vi "Save_current_setup.vi"(3 "Save New File?":bool, 5 "Folder":path) -> (0 "Cancelled?":bool, 1 "Saved filepath":path, 2 "Current Setup":path)   [LabVIEW 2010]
panel:
  in  "Cancel Button":bool
  in  "OK":bool
  out "Existing file names":string[](array[string])
  in  "New setup filename":string
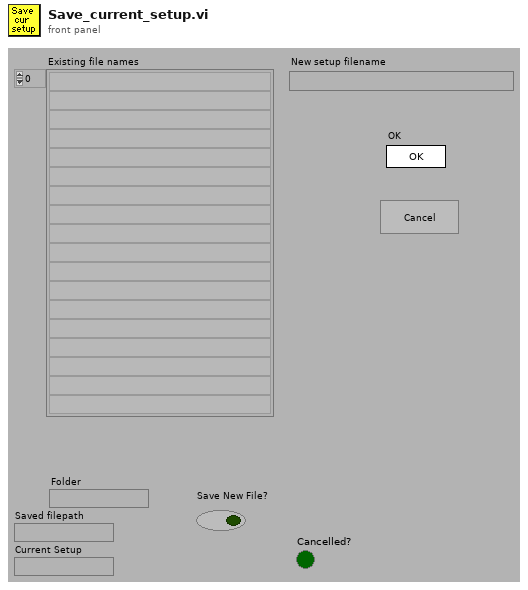
[diagram p1: front panel]
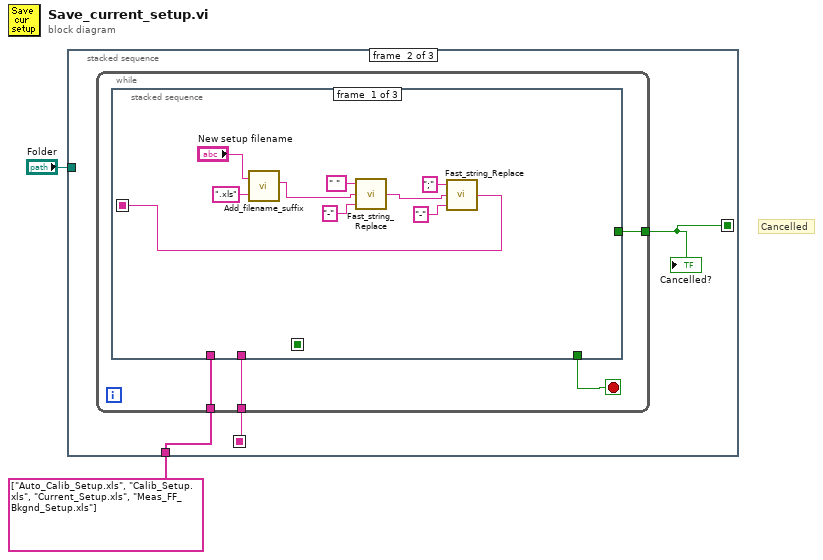
[diagram p0: block diagram]
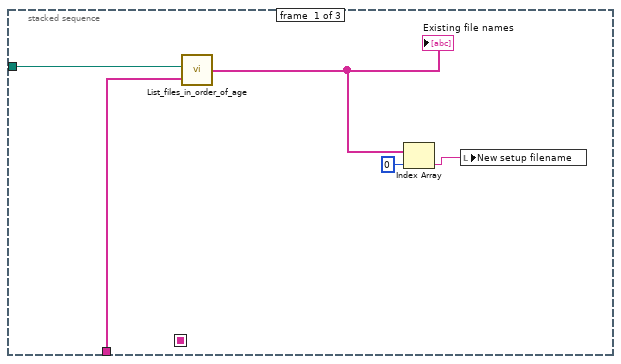
[diagram p2: hidden frame]
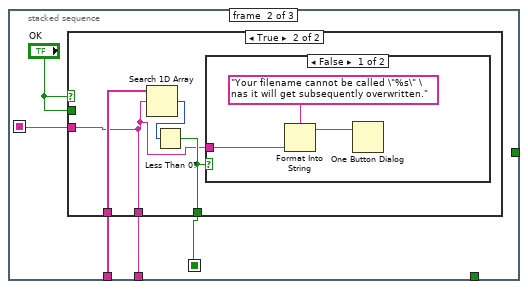
[diagram p3: hidden frame]
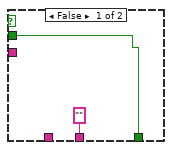
[diagram p4: hidden frame]
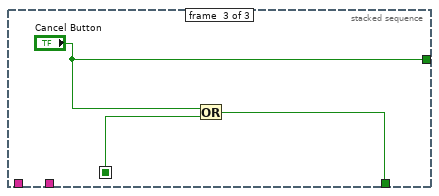
[diagram p6: hidden frame]
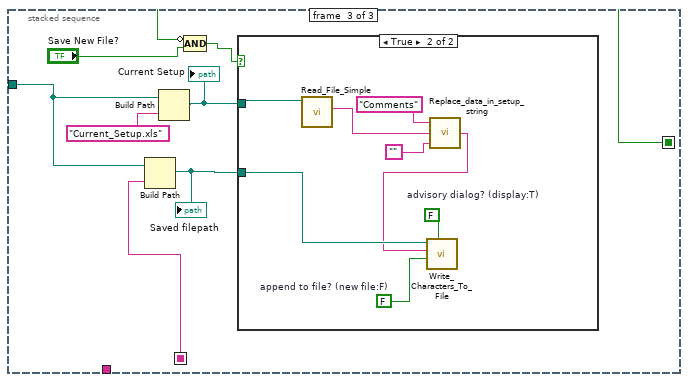
[diagram p7: hidden frame]
diagram:
  # "Cancelled"
  n1 = stacked-sequence {
    seq-local: [_ w10 _] -> [_ _ w47]
    seq-local: [_ w9 _] -> [_ _ w43]
    tunnel: "Folder" -> [w7 _ w46]
    tunnel: string[] ["Auto_Calib_Setup.xls", "Calib_Setup.xls", "Current_Setup.xls", "Meas_FF_Bkgnd_Setup.xls"] ("file names") -> [w6 w8 _]
    frame #0 {
      n2 = call "List_files_in_order_of_age.vi"("Files to Hide"=w6, "Folder"=w7) -> ("file names"=w5:string[])
      "Existing file names" <- w5
      n3 = Index Array(array=w5, index=0) -> (element=w3:string)
      n4 = local write "New setup filename"(w3) -> ()
    }
    frame #1 {
      n5 = while {
        tunnel: [w14] -> w10
        tunnel: [w12] -> w9
        tunnel: w8 -> [w11]
        stop <- w13 stop-if-true
        n6 = stacked-sequence {
          seq-local: [w15 _ _] -> [_ w28 _]
          seq-local: [_ w26 _] -> [_ _ w40]
          tunnel: [_ w27 _] -> w14
          tunnel: [_ _ w39] -> w13
          tunnel: [_ _ "Cancel Button"] -> w12
          tunnel: w11 -> [_ w24 _]
          frame #0 {
            n7 = call "Add_filename_suffix.vi"("Filename"="New setup filename", "Suffix to add"=".xls") -> ("Filename out"=w20:string)  [unwired: 3 out]
            n8 = call "Fast_string_Replace.vi"("Replace match with:"="-", "Input String"=w20, "regular expression"=" ") -> ("Output String"=w16:string)  [unwired: 2 out]
            n9 = call "Fast_string_Replace.vi"("Replace match with:"="-", "Input String"=w16, "regular expression"=";") -> ("Output String"=w15:string)  [unwired: 2 out]
          }
          frame #1 {
            n10 = case shown="True" "OK" {
              tunnel: w28 -> [_ w31]
              tunnel: [w29 w32] -> w26
              tunnel: ["" ("File name only") w31] -> w27
              tunnel: "OK" -> [w29 _]
              tunnel: w24 -> [_ w34]
              frame False {
              }
              frame True {
                n11 = Search 1D Array(1D array=w34, element=w31) -> (index of element=w33:i32)  [unwired: 1 out]
                n12 = Less Than 0?(x=w33) -> (x < 0?=w32:bool)
                n13 = case shown="False" w32 {
                  tunnel: w31 -> [w36 _]
                  frame False {
                    n14 = Format Into String(format string="Your filename cannot be called \"%s\" \nas it will get subsequently overwritten.", w36) -> (resulting string=w35:string)  [unwired: 2 in, 1 out]
                    n15 = One Button Dialog(message=w35) -> ()  [unwired: 2 out]
                  }
                  frame True {
                  }
                }
              }
            }
          }
          frame #2 {
            n16 = Or(x="Cancel Button", y=w40) -> (x .or. y?=w39:bool)
          }
        }
      }
      "Cancelled?" <- w9
    }
    frame #2 {
      n17 = Build Path(base path=w46, name or relative path=w47) -> (appended path=w44:path)
      "Saved filepath" <- w44
      n18 = Build Path(base path=w46, name or relative path="Current_Setup.xls") -> (appended path=w45:path)
      "Current Setup" <- w45
      n19 = Compound Arithmetic op=AND(invert w43, "Save New File?") -> (w41:bool)
      n20 = case shown="True" w41 {
        tunnel: w45 -> [_ w56]
        tunnel: w44 -> [_ w55]
        frame False {
        }
        frame True {
          w53 = FALSE  # advisory dialog? (display:T)
          w54 = FALSE  # append to file? (new file:F)
          n21 = call "Read_File_Simple.vi"("Filename"=w56) -> ("string"=w50:string)  [unwired: 2 in, 7 out]
          n22 = call "Replace_data_in_setup_string.vi"("New data string"="", "Input string"=w50, "Variable name"="Comments") -> ("Appended string"=w49:string)
          n23 = call "Write_Characters_To_File.vi"("file path (dialog if empty)"=w55, "advisory dialog? (display:T)"=w53, "character string"=w49, "append to file? (new file:F)"=w54) -> ()  [unwired: 1 in, 4 out]
        }
      }
    }
  }
